vi "Memory.Pointer.SGL.New.vi"(8 "error in (no error)":errorcluster, 11 "count (1)":u64 format="%d elements") -> (0 "error out":errorcluster, 3 "pointer":refnum<class "Memory.Pointer.SGL.lvclass">)   [LabVIEW 2016, in "Memory.lvlib" / "Memory.Pointer.SGL.lvclass"]
uses:
  Memory.Pointer.SGL.lvclass
  C:/Git/SourceTree/DSF/Source/Submodules/Memory/Source/Classes/Internal/Memory.Pointer.Internal.lvclass
  Internal/Memory.Pointer.Internal.lvclass
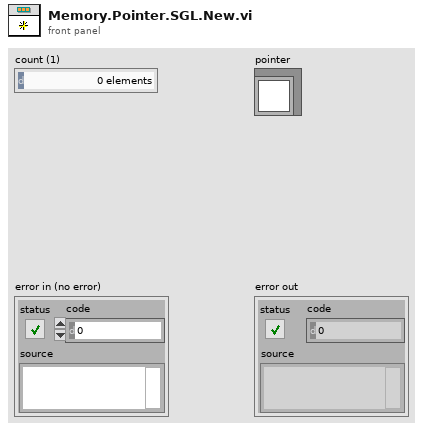
[diagram p1: front panel]
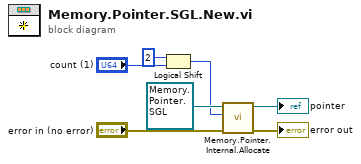
[diagram p0: block diagram]
diagram:
  n1 = Logical Shift(y=i16 2 ("power of 2"), x="count (1)") -> (x << y=w1:u64)
  n2 = call "Memory.Pointer.Internal.Allocate.vi"("error in (no error)"="error in (no error)", "size"=w1, "pointer in"=refnum<class "Memory.Pointer.SGL.lvclass"> refnum ("DBL Pointer")) -> ("error out"=→"error out":errorcluster, "pointer out"=→"pointer":refnum<class "Memory.Pointer.SGL.lvclass">)  [unwired: 7 in]
